vi "GetKey.vi"(8 "error in (no error)":errorcluster, 9 "PassWord":string, 10 "UserName":string(combo), 11 "UserManagement in":refnum<class "UserManagement.lvclass">) -> (0 "error out":errorcluster, 2 "LoginResponse":cluster{"UserInfo":T1, "PassWordExists？":bool}, 3 "UserManagement out":refnum<class "UserManagement.lvclass">)   [LabVIEW 2019, in "UserManagement.lvlib" / "UserManagement.lvclass"]
uses:
  UserManagement.lvclass
  UserInfo.ctl
  Permission.ctl
  UserManagement.lvclass/UserManagement.ctl
  <vilib>/Utility/config.llb/Read Key (String).vi
  <vilib>/Utility/config.llb/NI_LVConfig.lvlib
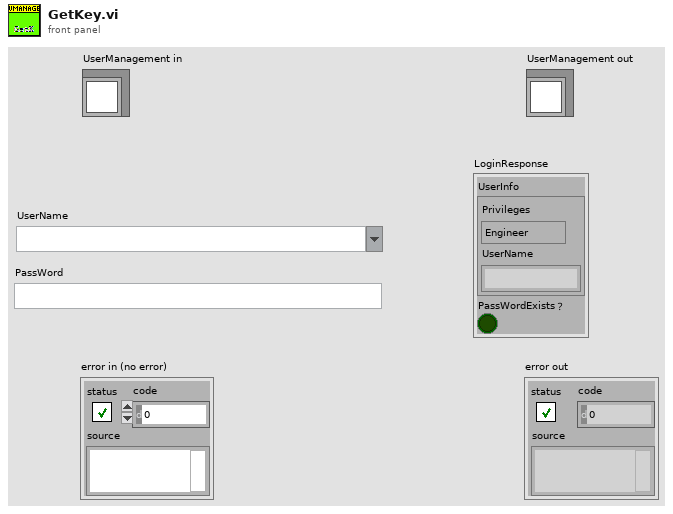
[diagram p1: front panel]
types:
  T1 = typedef "UserManagement.lvlib/UserManagement.lvclass/UserInfo.ctl" = cluster{"Privileges":T2, "UserName":string}
  T2 = typedef "UserManagement.lvlib/UserManagement.lvclass/Permission.ctl" = enum16{"Engineer", "Technical", "Operator"}
  T3 = typedef "NI_LVConfig.lvlib/Config Data RefNum.ctl" = refnum<k1>
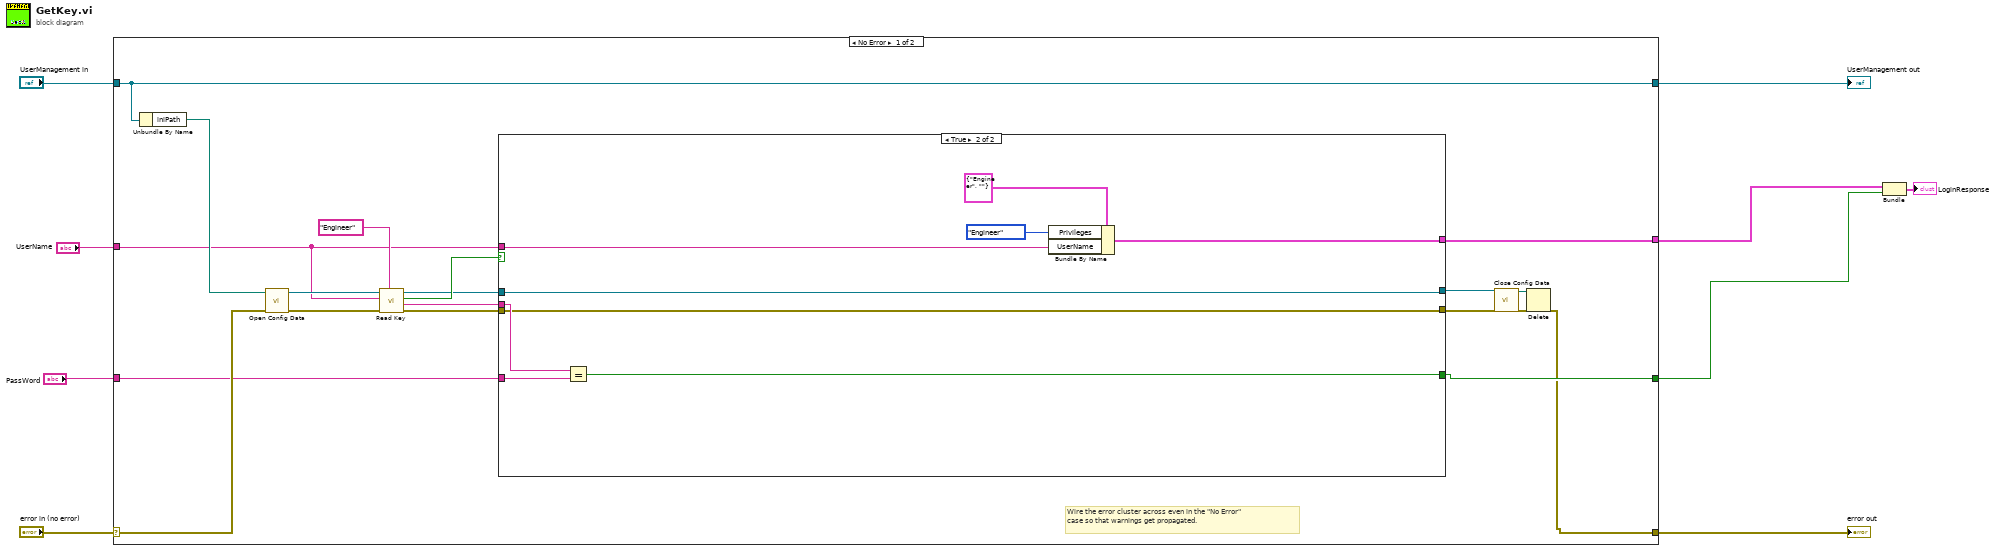
[diagram p0: block diagram]
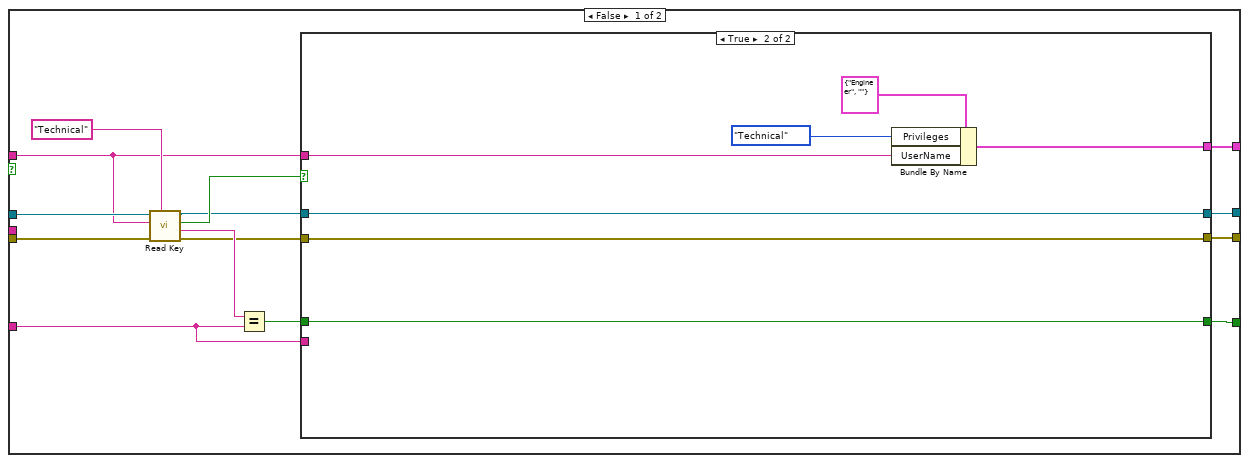
[diagram p2: hidden frame]
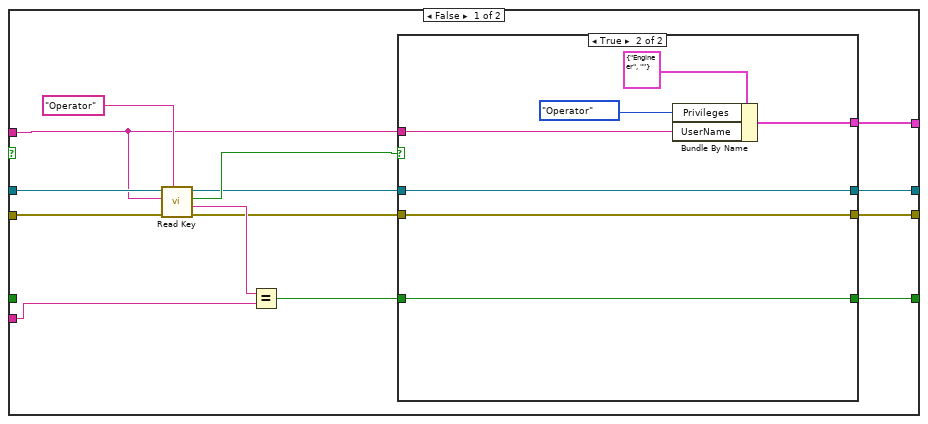
[diagram p3: hidden frame]
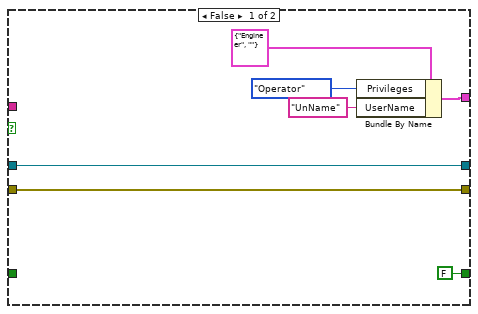
[diagram p4: hidden frame]
diagram:
  n1 = case shown="No Error" "error in (no error)" {
    selector: "error in (no error)" -> [w16 w88]
    tunnel: [w12 w88] -> w8
    tunnel: [w11 w87] -> w6
    tunnel: "UserManagement in" -> [w11 w87]
    tunnel: "UserName" -> [w15 _]
    tunnel: "PassWord" -> [w14 _]
    tunnel: [w13 _] -> w2
    tunnel: [w10 _] -> w3
    frame No Error {
      # "Wire the error cluster across even in the \"No Error\"\ncase so that warnings get propagated."
      n2 = Unbundle By Name(w11) -> ("iniPath"=w17:path)
      n3 = call <vilib>:"Open Config Data.vi"("error in (no error)"=w16, "configuration file path"=w17) -> ("error out"=w27:errorcluster, "refnum"=w28:T3)  [unwired: 7 in, 1 out]
      n4 = call-poly <vilib>:"Read Key.vi"("section"="Engineer", "error in (no error)"=w27, "key"=w15, "refnum"=w28) -> ("error out"=w26:errorcluster, "value"=w23:string, "found?"=w25:bool, "refnum out"=w24:T3)  [unwired: 4 in]
      n5 = case shown="True" w25 {
        tunnel: w26 -> [w41 w81]
        tunnel: w24 -> [w42 w80]
        tunnel: w23 -> [_ w86]
        tunnel: w14 -> [w33 w85]
        tunnel: [w37 w84] -> w13
        tunnel: w15 -> [w29 w83]
        tunnel: [w35 w82] -> w10
        tunnel: [w32 w81] -> w19
        tunnel: [w31 w80] -> w18
        frame False {
          n6 = call-poly <vilib>:"Read Key.vi"("section"="Technical", "error in (no error)"=w41, "key"=w29, "refnum"=w42) -> ("error out"=w38:errorcluster, "value"=w39:string, "found?"=w40:bool, "refnum out"=w34:T3)  [unwired: 4 in]
          n7 = Equal?(x=w39, y=w33) -> (x = y?=w36:bool)
          n8 = case shown="True" w40 {
            tunnel: w38 -> [w55 w74]
            tunnel: [w52 w77] -> w37
            tunnel: w36 -> [_ w77]
            tunnel: w29 -> [w43 w76]
            tunnel: [w49 w75] -> w35
            tunnel: w34 -> [w54 w73]
            tunnel: w33 -> [w53 _]
            tunnel: [w47 w74] -> w32
            tunnel: [w45 w73] -> w31
            frame False {
              n9 = call-poly <vilib>:"Read Key.vi"("section"="Operator", "error in (no error)"=w55, "key"=w43, "refnum"=w54) -> ("error out"=w48:errorcluster, "value"=w56:string, "found?"=w50:bool, "refnum out"=w46:T3)  [unwired: 4 in]
              n10 = Equal?(x=w56, y=w53) -> (x = y?=w51:bool)
              n11 = case shown="True" w50 {
                tunnel: [FALSE w70] -> w52
                tunnel: w51 -> [_ w70]
                tunnel: w43 -> [_ w69]
                tunnel: [w62 w68] -> w49
                tunnel: [w63 w67] -> w47
                tunnel: w48 -> [w63 w67]
                tunnel: w46 -> [w60 w66]
                tunnel: [w60 w66] -> w45
                frame False {
                  n12 = Bundle By Name(cluster=T1 {"Privileges"=enum."Engineer", "UserName"=""} ("UserInfo"), "Privileges"=Permission."Operator" ("Permission"), "UserName"="UnName") -> (w62:T1)
                }
                frame True {
                  n13 = Bundle By Name(cluster=T1 {"Privileges"=enum."Engineer", "UserName"=""} ("UserInfo"), "Privileges"=Permission."Operator" ("Permission"), "UserName"=w69) -> (w68:T1)
                }
              }
            }
            frame True {
              n14 = Bundle By Name(cluster=T1 {"Privileges"=enum."Engineer", "UserName"=""} ("UserInfo"), "Privileges"=Permission."Technical" ("Permission"), "UserName"=w76) -> (w75:T1)
            }
          }
        }
        frame True {
          n15 = Equal?(x=w86, y=w85) -> (x = y?=w84:bool)
          n16 = Bundle By Name(cluster=T1 {"Privileges"=enum."Engineer", "UserName"=""} ("UserInfo"), "Privileges"=Permission."Engineer" ("Permission"), "UserName"=w83) -> (w82:T1)
        }
      }
      n17 = call <vilib>:"Close Config Data.vi"("error in (no error)"=w19, "refnum"=w18) -> ("error out"=w21:errorcluster, "file path"=w20:path)  [unwired: 8 in]
      n18 = Delete(path (use dialog)=w20, error in=w21) -> (error out=w12:errorcluster)  [unwired: 3 in, 2 out]
    }
    frame Error {
    }
  }
  "error out" <- w8
  "UserManagement out" <- w6
  n19 = Bundle("UserInfo"=w3, w2) -> (→"LoginResponse":cluster{"UserInfo":T1, bool})  [unwired: 1 in]
